vi "Read Single.vi"   [LabVIEW 2012, in "NH Research Regenerative Test Series.lvlib"]
doc: "Initiates and reads a single measurement."
uses:
  <instrlib>/NH Research Regenerative Test Series/NH Research Regenerative Test Series.lvlib
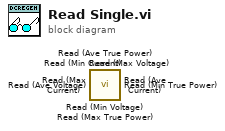
[diagram p0: block diagram]
diagram:
  n1 = call <instrlib>:"Read (Min Voltage).vi"() -> ()  [unwired: 13 in, 3 out]
  n2 = call <instrlib>:"Read (Max Voltage).vi"() -> ()  [unwired: 13 in, 3 out]
  n3 = call <instrlib>:"Read (Ave Voltage).vi"() -> ()  [unwired: 13 in, 3 out]
  n4 = call <instrlib>:"Read (Min True Power).vi"() -> ()  [unwired: 13 in, 3 out]
  n5 = call <instrlib>:"Read (Max True Power).vi"() -> ()  [unwired: 13 in, 3 out]
  n6 = call <instrlib>:"Read (Ave True Power).vi"() -> ()  [unwired: 13 in, 3 out]
  n7 = call <instrlib>:"Read (Min Current).vi"() -> ()  [unwired: 13 in, 3 out]
  n8 = call <instrlib>:"Read (Max Current).vi"() -> ()  [unwired: 13 in, 3 out]
  n9 = call <instrlib>:"Read (Ave Current).vi"() -> ()  [unwired: 13 in, 3 out]
